vi "NFL_L_bank_Control_07.vi"(0 "SI804.lvclass in":refnum<class "SI804.lvclass">, 1 "3 JSA20 DT109\nXA01":bool, 2 "3 JSA20 DT108\nXA01":bool, 3 "3 JSA20 DT110\nXA01":bool, 5 "error in":errorcluster, 6 "ACT-Ctrl\nL-bank insertion":bool, 7 "ACT-Ctrl\nL-bank withdrawal":bool) -> (14 "SI804.lvclass out":refnum<class "SI804.lvclass">, 15 "L-bank ins":bool, 16 "NFL-Control M/A":bool, 17 "L-bank withdr":bool, 19 "error out":errorcluster)   [LabVIEW 2022 SP3, in "SI804.lvclass"]
uses:
  SI804.lvclass
  SI804.lvclass/SI804.ctl
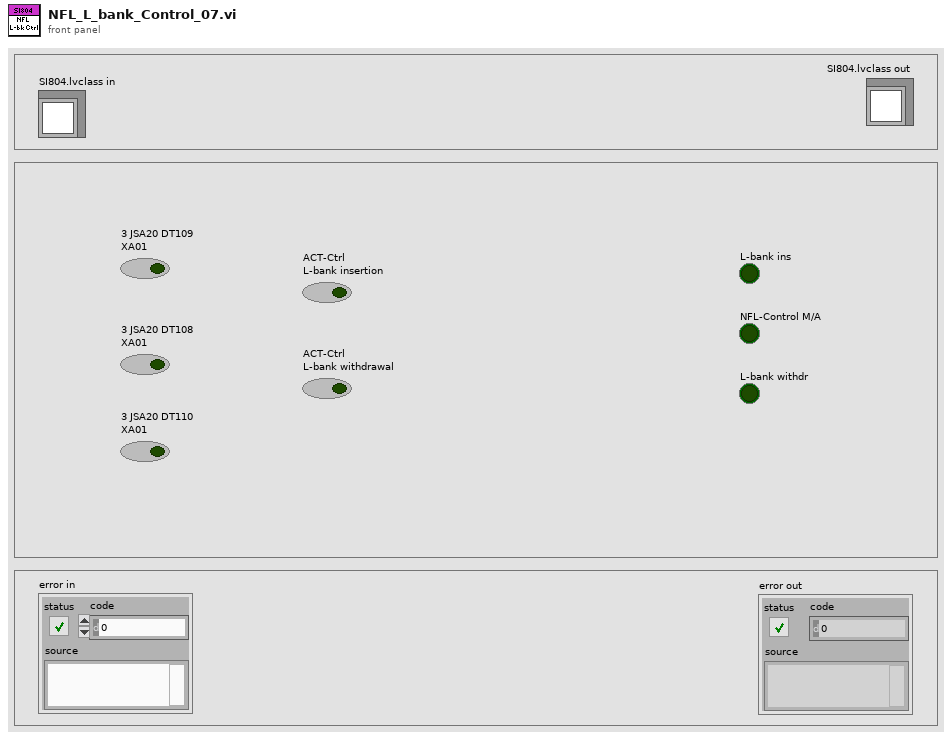
[diagram p1: front panel]
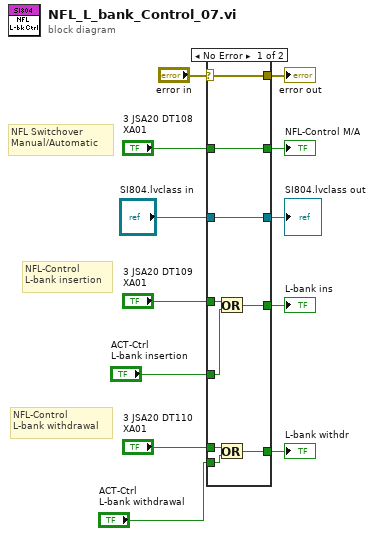
[diagram p0: block diagram]
diagram:
  # "NFL-Control\nL-bank withdrawal"
  # "NFL Switchover\nManual/Automatic"
  # "NFL-Control\nL-bank insertion"
  n1 = case shown="No Error" "error in" {
    selector: "error in" -> [w13 w22]
    tunnel: "3 JSA20 DT109\nXA01" -> [w20 _]
    tunnel: "3 JSA20 DT108\nXA01" -> [w17 _]
    tunnel: "3 JSA20 DT110\nXA01" -> [w19 _]
    tunnel: "SI804.lvclass in" -> [w14 w23]
    tunnel: "ACT-Ctrl\nL-bank insertion" -> [w21 _]
    tunnel: "ACT-Ctrl\nL-bank withdrawal" -> [w18 _]
    tunnel: [w17 _] -> w4
    tunnel: [w16 _] -> w5
    tunnel: [w15 _] -> w3
    tunnel: [w14 w23] -> w2
    tunnel: [w13 w22] -> w1
    frame No Error {
      n2 = Or(x=w20, y=w21) -> (x .or. y?=w16:bool)
      n3 = Or(x=w19, y=w18) -> (x .or. y?=w15:bool)
    }
    frame Error {
    }
  }
  "L-bank ins" <- w5
  "NFL-Control M/A" <- w4
  "L-bank withdr" <- w3
  "SI804.lvclass out" <- w2
  "error out" <- w1
